vi "Main VI w_o ring.vi"() -> ()   [LabVIEW 2017]
uses:
  data.ctl
  caseConstrol.ctl
  data cluster.ctl
  <vilib>/Instr/_visa.llb/VISA Configure Serial Port (Instr).vi
  <vilib>/Analysis/3filter.llb/Butterworth Filter (DBL).vi
  <vilib>/Analysis/NI_AALBase.lvlib
panel:
  out "Index Volt":string
  out "Thumb Volt":string
  out "Waveform Chart":dbl[](graph)
  in  "Stop Button":bool
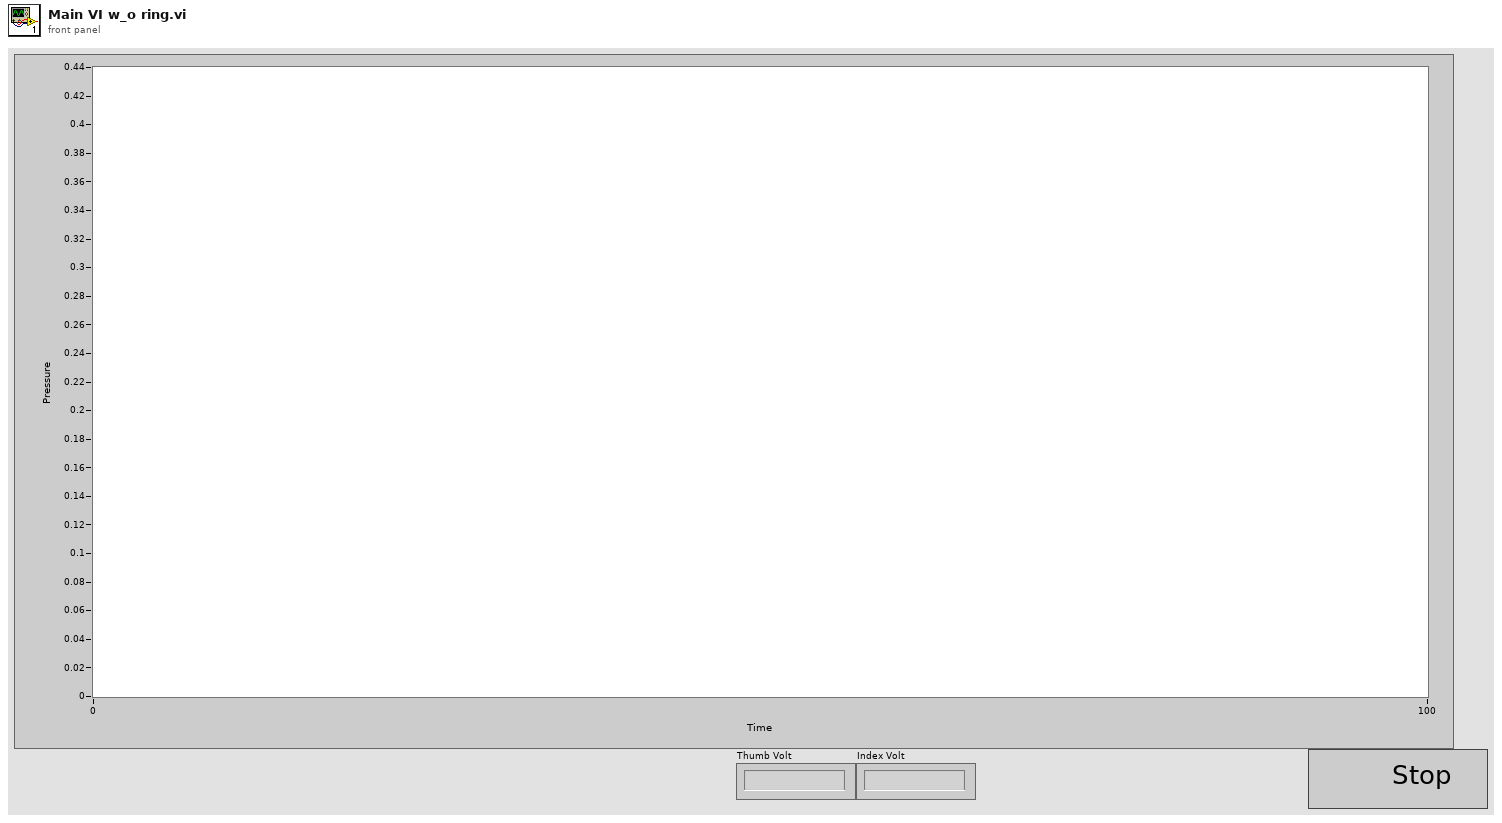
[diagram p1: front panel]
types:
  T1 = typedef "data cluster.ctl" = cluster{"Pressure":dbl[], "Waveform":waveform(dbl), "Voltage":dbl[]}
  T2 = enum16{"open", "replace", "create", "open or create", "replace or create", "replace or create with confirmation"}
  T3 = typedef "caseConstrol.ctl" = enum16{"Initialize", "Wait for Event", "Convert Signal", "Noise Processing", "Threshold Processing", "Stop"}
  T4 = typedef "data.ctl" = cluster{"First Name:":string, "Last Name:":string, "Threshold Number:":dbl}
  T5 = cluster{"First Name:":string, "Last Name:":string, "Threshold number:":dbl}
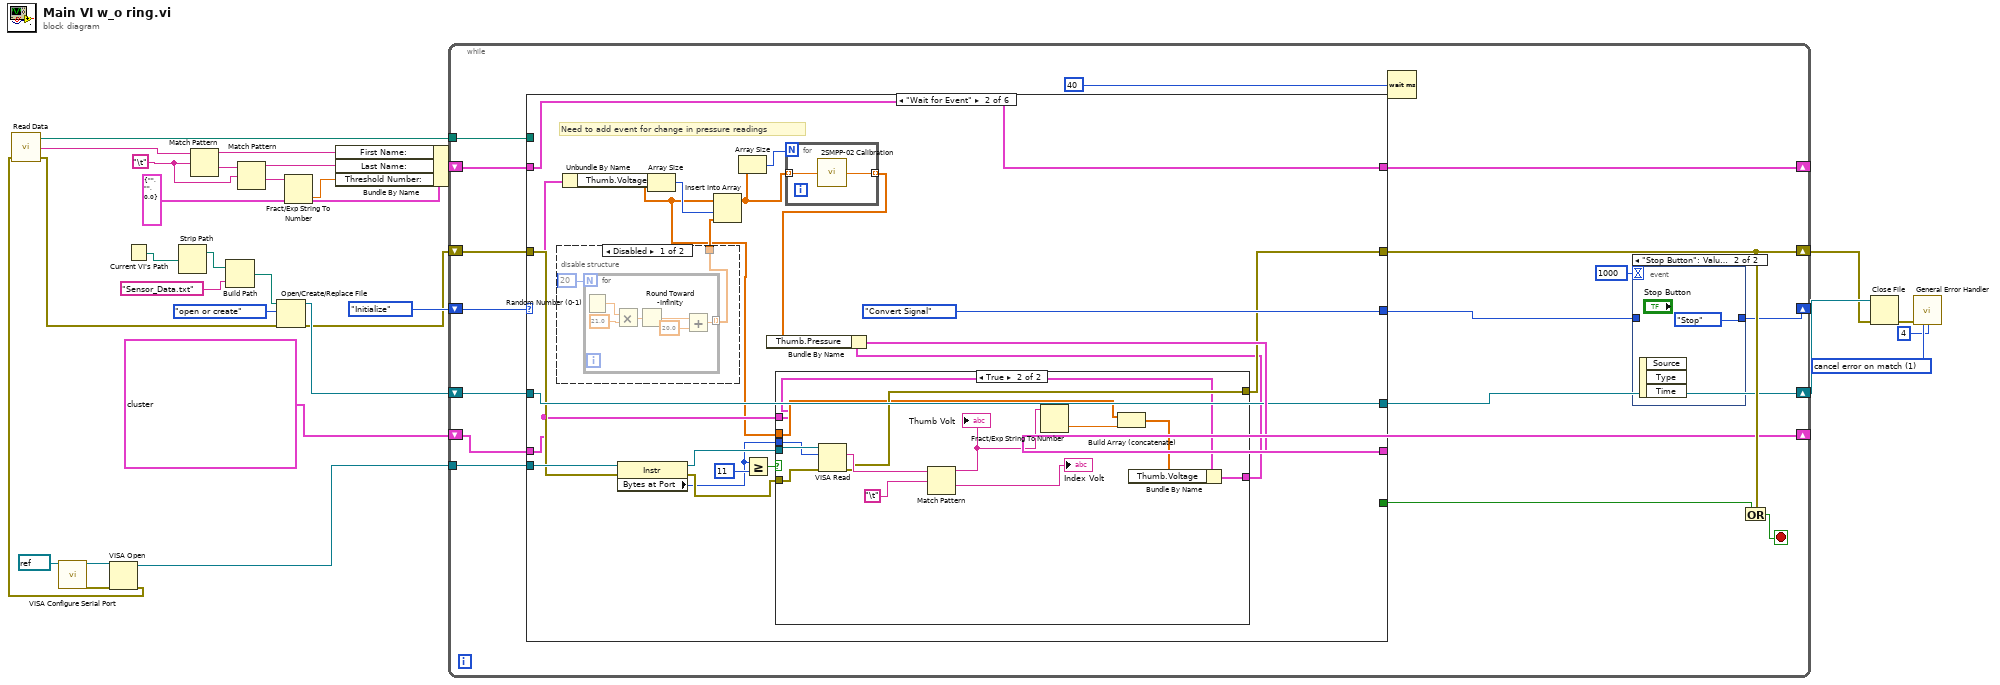
[diagram p0: block diagram]
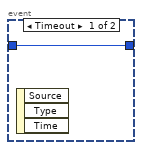
[diagram p2: hidden frame]
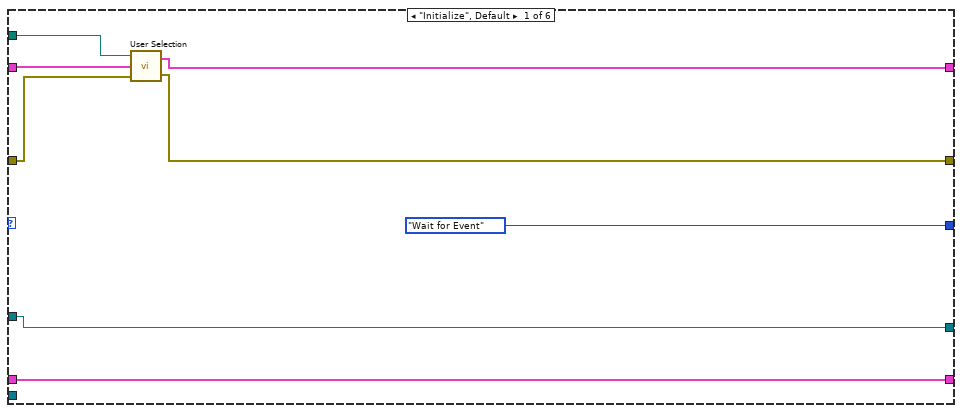
[diagram p3: hidden frame]
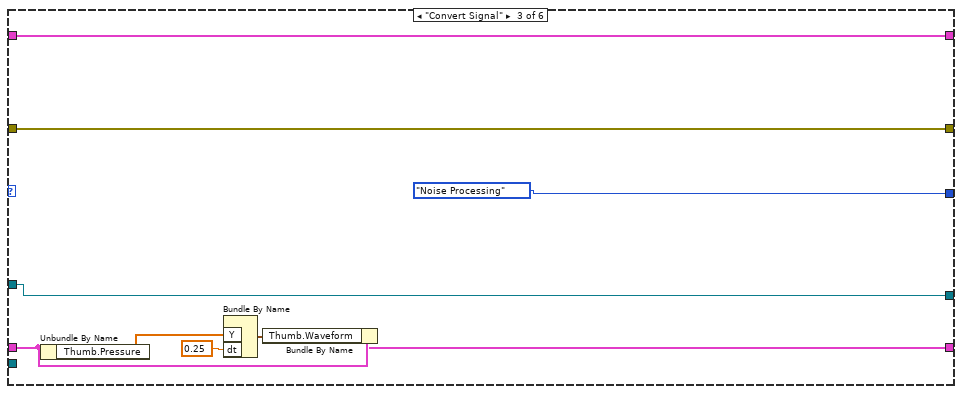
[diagram p6: hidden frame]
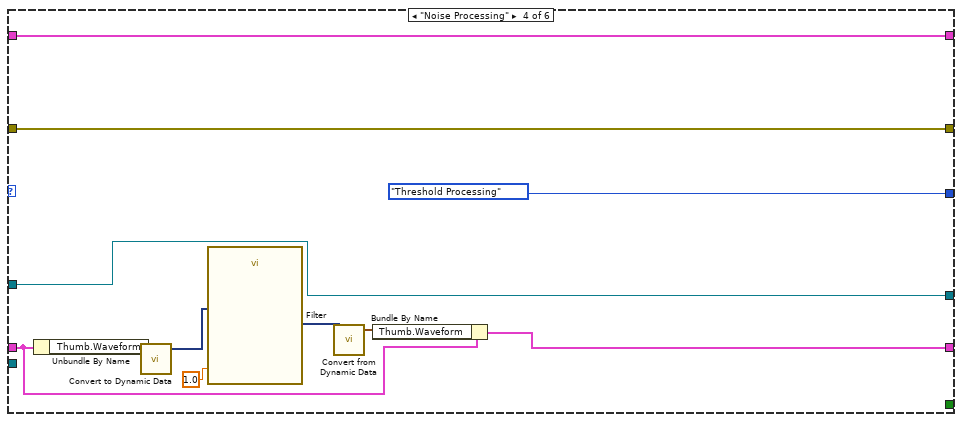
[diagram p7: hidden frame]
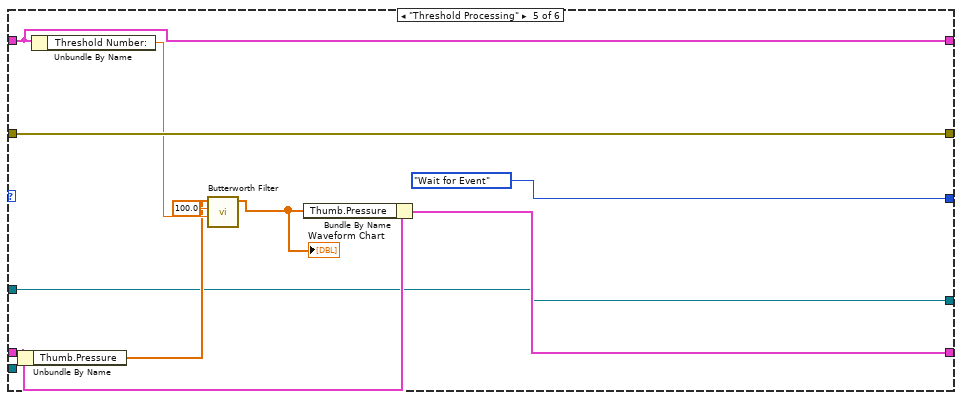
[diagram p8: hidden frame]
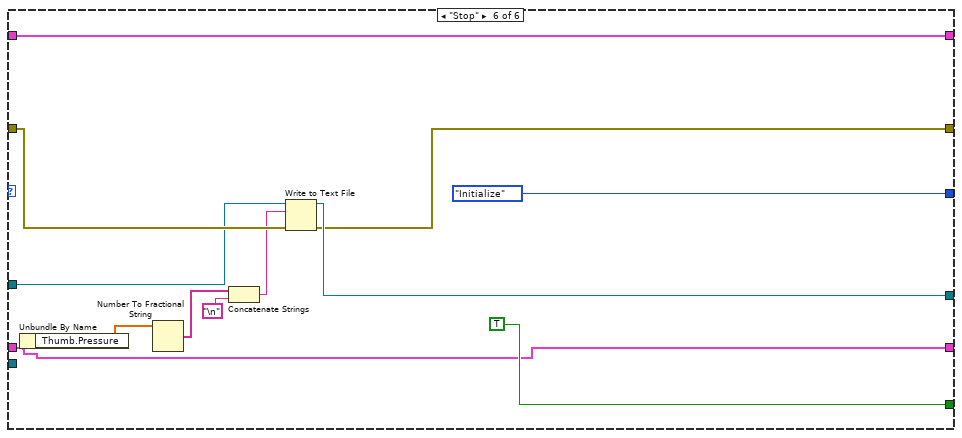
[diagram p9: hidden frame]
diagram:
  w12 = 1 items=["no exception", "cancel error on match", "set error on match"] ("[exception action] (none:0)")
  w29 = "\t"
  n1 = call-poly "VISA Configure Serial Port"("VISA resource name"=refnum<visa-resource-name> refnum) -> ("VISA resource name out"=w4:refnum<visa-resource-name>, "error out"=w5:errorcluster)  [unwired: 13 in]
  n2 = VISA Open(error in (no error)=w5, VISA resource name=w4) -> (VISA resource name=w3:refnum<visa-resource-name>, error out=w2:errorcluster)  [unwired: 3 in]
  n3 = call "Read Data.vi"("Error In"=w2) -> ("error out"=w17:errorcluster, "text"=w26:string, "appended path"=w25:path)  [unwired: 2 in]
  n4 = Current VI's Path() -> (path=w10:path)
  n5 = Strip Path(path=w10) -> (stripped path=w9:path)  [unwired: 1 out]
  n6 = Match Pattern(string=w26, regular expression=w29) -> (before substring=w20:string, after substring=w30:string)  [unwired: 1 in, 2 out]
  n7 = Build Path(base path=w9, name or relative path="Sensor_Data.txt") -> (appended path=w7:path)
  n8 = Match Pattern(string=w30, regular expression=w29) -> (before substring=w21:string, after substring=w28:string)  [unwired: 1 in, 2 out]
  n9 = Open/Create/Replace File(file path (use dialog)=w7, error in=w17, operation (0:open)=T2."open or create") -> (refnum out=w18:refnum<file>, error out=w16:errorcluster)  [unwired: 3 in, 1 out]
  n10 = Fract/Exp String To Number(string=w28) -> (number=w22:dbl)  [unwired: 3 in, 1 out]
  n11 = Bundle By Name(cluster=T4 {"First Name:"="", "Last Name:"="", "Threshold Number:"=0.0}, "First Name:"=w20, "Last Name:"=w21, "Threshold Number:"=w22) -> (w23:T4)
  n12 = while {
    shift-right: [w43] -> _
    shift-left: w23 -> [w46]
    shift-right: [w37] -> _
    shift-left: caseConstrol."Initialize" -> [w47]
    tunnel: w25 -> [w44]
    shift-right: [w40] -> w14
    shift-left: w16 -> [w45]
    shift-right: [w33] -> w15
    shift-left: w18 -> [w36]
    shift-right: [w34] -> _
    shift-left: cluster{"Thumb":T1, "Index":T1} {"Thumb"={"Pressure"=[], "Waveform"={"t0"=timestamp(0 s since 1904-01-01), "dt"=1.0, "Y"=[]}, "Voltage"=[]}, "Index"={"Pressure"=[], "Waveform"={"t0"=timestamp(0 s since 1904-01-01), "dt"=1.0, "Y"=[]}, "Voltage"=[]}} -> [w35]
    tunnel: w3 -> [w31]
    stop <- w41 stop-if-true
    n13 = case shown="\"Wait for Event\"" w47 {
      tunnel: [_ _ _ _ _ TRUE] -> w42
      tunnel: w46 -> [w57 w75 w110 w120 w123 w143]
      tunnel: w45 -> [w56 w68 w111 w121 w131 w139]
      tunnel: w44 -> [w55 _ _ _ _ _]
      tunnel: [caseConstrol."Wait for Event" caseConstrol."Convert Signal" caseConstrol."Noise Processing" caseConstrol."Threshold Processing" caseConstrol."Wait for Event" caseConstrol."Initialize"] -> w38
      tunnel: [w53 w75 w110 w120 w123 w143] -> w43
      tunnel: [w52 w62 w111 w121 w131 w136] -> w40
      tunnel: w36 -> [w50 w70 w103 w113 w125 w138]
      tunnel: [w51 w71 w104 w112 w126 w133] -> w34
      tunnel: w35 -> [w51 w61 w105 w115 w127 w133]
      tunnel: [w50 w70 w103 w113 w125 w137] -> w33
      tunnel: w31 -> [_ w69 _ _ _ _]
      frame "Initialize", Default {
        n14 = call "User Selection.vi"("error in (no error)"=w56, "Cluster"=w57, "file path (use dialog)"=w55) -> ("error out"=w52:errorcluster, "Cluster 2"=w53:T5)
      }
      frame "Wait for Event" {
        # "Need to add event for change in pressure readings"
        n15 = disable-structure shown="Disabled" {
          disable-tunnel: [w78 _] -> w73
          frame Disabled {
            n16 = for {
              N: 20 -> [_]
              tunnel: [w80] -> w78 mode=indexing
              n17 = Random Number (0-1)() -> (number: 0 to 1=w85:dbl)
              n18 = Multiply(x=w85, y=21.0) -> (x*y=w83:dbl)
              n19 = Round Toward -Infinity(1:w83) -> (0:w82:dbl)
              n20 = Add(x=w82, y=20.0) -> (x+y=w80:dbl)
            }
          }
          frame Enabled {
          }
        }
        n21 = Unbundle By Name(w61) -> ("Thumb.Voltage"=w59:dbl[])
        n22 = property class="Instr"(reference=w69, error in=w68) -> (reference out=w65:refnum<visa-resource-name>, error out=w64:errorcluster, "Bytes at Port"=w63:u32)
        n23 = Array Size(array=w59) -> (size(s)=w74:i32)
        n24 = Insert Into Array(array=w59, index=w74, new element=w73) -> (w60:dbl[])
        n25 = Array Size(array=w60) -> (size(s)=w72:i32)
        n26 = Greater Or Equal?(x=w63, y=u32 11) -> (x >= y?=w67:bool)
        n27 = case shown="True" w67 {
          tunnel: w65 -> [_ w99]
          tunnel: w64 -> [w87 w100]
          tunnel: w63 -> [_ w98]
          tunnel: [w87 w95] -> w62
          tunnel: w61 -> [w86 w90]
          tunnel: w59 -> [_ w93]
          tunnel: [w86 w89] -> w58
          frame False {
          }
          frame True {
            n28 = VISA Read(VISA resource name=w99, byte count=w98, error in (no error)=w100) -> (read buffer=w97:string, error out=w95:errorcluster)  [unwired: 2 out]
            n29 = Match Pattern(string=w97, regular expression="\t") -> (before substring=w94:string, after substring=→"Index Volt":string)  [unwired: 1 in, 2 out]
            "Thumb Volt" <- w94
            n30 = Fract/Exp String To Number(string=w94) -> (number=w92:dbl)  [unwired: 3 in, 1 out]
            n31 = Build Array (concatenate)(w93, w92) -> (w91:dbl[])
            n32 = Bundle By Name(cluster=w90, "Thumb.Voltage"=w91) -> (w89:cluster{"Thumb":T1, "Index":T1})
          }
        }
        n33 = for {
          N: w72 -> [_]
          tunnel: [w102] -> w76 mode=indexing
          tunnel: w60 -> [w101] mode=indexing
          n34 = call "2SMPP-02 Calibration.vi"("Sensor Voltage"=w101) -> ("Pressure"=w102:dbl)
        }
        n35 = Bundle By Name(cluster=w58, "Thumb.Pressure"=w76) -> (w71:cluster{"Thumb":T1, "Index":T1})
      }
      frame "Convert Signal" {
        n36 = Unbundle By Name(w105) -> ("Thumb.Pressure"=w107:dbl[])
        n37 = Bundle By Name("Y"=w107, "dt"=0.25) -> (w106:waveform(dbl))  [unwired: 1 in]
        n38 = Bundle By Name(cluster=w105, "Thumb.Waveform"=w106) -> (w104:cluster{"Thumb":T1, "Index":T1})
      }
      frame "Noise Processing" {
        n39 = Unbundle By Name(w115) -> ("Thumb.Waveform"=w119:waveform(dbl))
        n40 = call "Convert to Dynamic Data"("Waveform"=w119) -> ("Dynamic Data Type"=w118:dynamicdata)  [unwired: 3 in]
        n41 = call "Filter"("Lower Cut-Off"=1.0, "Signal"=w118) -> ("Filtered Signal"=w116:dynamicdata)  [unwired: 8 in, 1 out]
        n42 = call "Convert from Dynamic Data"("Dynamic Data Type"=w116) -> ("Waveform"=w114:waveform(dbl))  [unwired: 3 in]
        n43 = Bundle By Name(cluster=w115, "Thumb.Waveform"=w114) -> (w112:cluster{"Thumb":T1, "Index":T1})
      }
      frame "Threshold Processing" {
        n44 = Unbundle By Name(w127) -> ("Thumb.Pressure"=w128:dbl[])
        n45 = Unbundle By Name(w123) -> ("Threshold Number:"=w130:dbl)
        n46 = call-poly <vilib>:"Butterworth Filter.vi"("high cutoff freq: fh"=w130, "sampling freq: fs"=100.0, "X"=w128) -> ("Filtered X"=w124:dbl[])  [unwired: 5 in, 1 out]
        "Waveform Chart" <- w124
        n47 = Bundle By Name(cluster=w127, "Thumb.Pressure"=w124) -> (w126:cluster{"Thumb":T1, "Index":T1})
      }
      frame "Stop" {
        n48 = Unbundle By Name(w133) -> ("Thumb.Pressure"=w141:dbl[])
        n49 = Number To Fractional String(number=w141) -> (F-format string=w140:string[])  [unwired: 3 in]
        n50 = Concatenate Strings(w140, "\n") -> (w134:string)
        n51 = Write to Text File(file (use dialog)=w138, text=w134, error in=w139) -> (refnum out=w137:refnum<file>, error out=w136:errorcluster)  [unwired: 1 in, 1 out]
      }
    }
    n52 = Wait (ms)(milliseconds to wait=u32 40) -> ()  [unwired: 1 out]
    n53 = event shown="[1] \"Stop Button\": Value Change" {
      selector: _ -> [_ _]
      dyn-events: _ -> [_ _]
      timeout: 1000 -> [_ _]
      tunnel: w38 -> [w48 _]
      tunnel: [w48 caseConstrol."Stop"] -> w37
      event Timeout {
        n54 = event-data() -> ()  [unwired: 1 in, 3 out]
      }
      event "Stop Button": Value Change {
        n55 = event-data() -> ()  [unwired: 1 in, 3 out]
      }
    }
    n56 = Or(x=w40, y=w42) -> (x .or. y?=w41:bool)
  }
  n57 = Close File(refnum=w15, error in=w14) -> (error out=w13:errorcluster)  [unwired: 1 out]
  n58 = call <vilib>:"General Error Handler.vi"("error in (no error)"=w13, "[exception action] (none:0)"=w12, "[exception code]"=4) -> ()  [unwired: 8 in, 5 out]
